vi "Control Type.vi"(11 "PulsedValve in":refnum<class "PulsedControl.lvclass">) -> (2 "Valve Type":string)   [LabVIEW 2020, in "VolatusControl.lvlib" / "PulsedControl.lvclass"]
uses:
  PulsedControl.lvclass
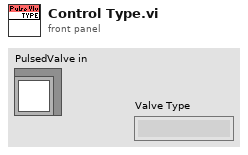
[diagram p1: front panel]
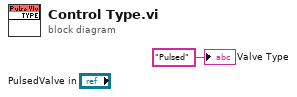
[diagram p0: block diagram]
diagram:
  "Valve Type" <- "Pulsed" ("Valve Type")
